vi "Periodic Tasks.vi"(8 "error in":errorcluster) -> ()   [LabVIEW 2015]
doc: "This VI runs in parallel to other tasks. It can contain as many user-defined periodic loops as you need. These can carry out PID or other sorts of timed response."
uses:
  ArmController/Typedef/ArmRef.ctl
  <vilib>/Rock Robotics/WPI/Potentiometer/WPI_PotentiometerDevRef.ctl
  <vilib>/Rock Robotics/SystemInterfaces/AI/FPGA_AIChannel.ctl
  <vilib>/Rock Robotics/WPI/MotorControl/WPI_MotorControlDeviceRef.ctl
  <vilib>/Rock Robotics/WPI/MotorControl/WPI_MotorControlType.ctl
  <vilib>/Rock Robotics/SystemInterfaces/DIO/FPGA_DIOPWMChannel.ctl
  <vilib>/Rock Robotics/WPI/PWM/WPI_PWMDeadband.ctl
  <vilib>/Rock Robotics/WPI/CAN/Jaguar/SubVIs/WPI_CANJaguar_ControlMode.ctl
  <vilib>/Rock Robotics/WPI/CAN/TalonSRX/WPI_CANTalonSRX_APIControlMode.ctl
  ArmController/Typedef/MessageType.ctl
  <vilib>/Rock Robotics/WPI/RobotDrive/WPI_RobotDriveDevRef.ctl
  Typedef/IntakeControllerMsg.ctl
  Typedef/IntakeControllerActions.ctl
  <vilib>/Rock Robotics/WPI/Utilities/WPI_GetSetVariantRefNum.vi
  <vilib>/Rock Robotics/WPI/Power/WPI_Power Get 5Volt Rail Voltage and Current.vi
  <vilib>/Rock Robotics/Network Tables/NT Write Number.vi
  ArmController/ArmController.lvlib
  NavX/navX Library v2.lvlib
panel:
  out "Logger timeout":bool
  out "# elements in Log queue":i32
  in  "Watts Rear":dbl=250.0 format="%#_13g"
  in  "Watts":dbl=320.0 format="%#_13g"
  out "Active Action":string
  in  "?":T1(tab)
  out "Motor Currents":T2(graph)
  out "Motor Power":T3(graph)
  out "Motor Voltage":dbl(graph)
  out "Pressure (psi)":dbl
  out "Pressure":dbl(graph)
  # "Competition: 320"
  # "Competition: 250"
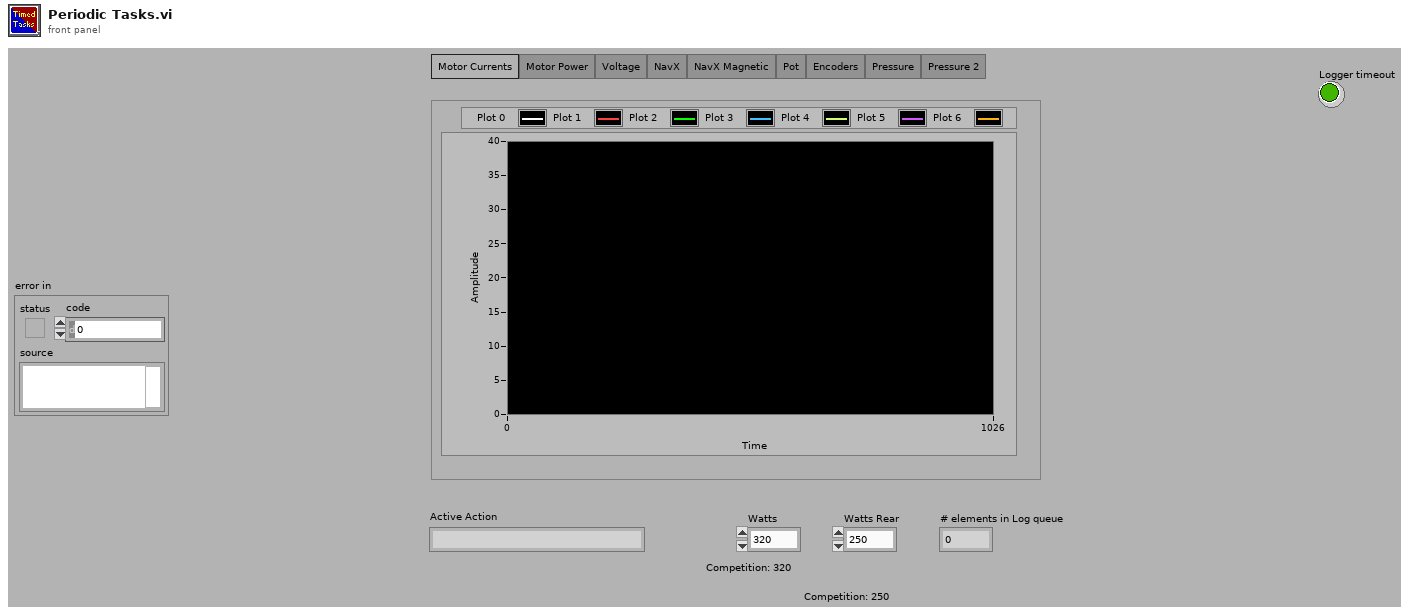
[diagram p1: front panel]
types:
  T1 = enum32{"Motor Currents", "Motor Power", "Voltage", "NavX", "NavX Magnetic", "Pot", "Encoders", "Pressure", "Pressure 2"}
  T2 = cluster{"all currents (A)[0]":dbl, "all currents (A)[1]":dbl, "all currents (A)[2]":dbl, "all currents (A)[3]":dbl, "all currents (A)[4]":dbl, "all currents (A)[5]":dbl, "all currents (A)[6]":dbl, "all currents (A)[7]":dbl, "all currents (A)[8]":dbl, "all currents (A)[9]":dbl, "all currents (A)[10]":dbl, "all currents (A)[11]":dbl, "all currents (A)[12]":dbl, "all currents (A)[13]":dbl}
  T3 = cluster{"[0]":dbl, "[1]":dbl, "[2]":dbl, "[3]":dbl, "[4]":dbl, "[5]":dbl, "[6]":dbl, "[7]":dbl, "[8]":dbl, "[9]":dbl, "[10]":dbl, "[11]":dbl, "[12]":dbl, "[13]":dbl}
  T4 = typedef "ArmController.lvlib/ArmRef.ctl" = cluster{"Pot":T5, "ArmMotor":T7, "Queue":refnum<queue>, "Setpoint":dbl, "Manual":bool, "output range":cluster{"output high":dbl, "output low":dbl}, "PID gains":cluster{"proportional gain (Kc)":dbl, "integral time (Ti, min)":dbl, "derivative time (Td, min)":dbl}}
  T5 = typedef "WPI_PotentiometerDevRef.ctl" = cluster{"DevStatus":errorcluster, "Analog Channel":T6, "Invert Output":bool}
  T6 = typedef "FPGA_AIChannel.ctl" = enum8{"AI 0", "AI 1", "AI 2", "AI 3", "AI MXP 0", "AI MXP 1", "AI MXP 2", "AI MXP 3", "Invalid"}
  T7 = typedef "WPI_MotorControlDeviceRef.ctl" = cluster{"DeviceStatus":errorcluster, "Type":T8, "PWM":cluster{"PWM Channel":T9, "DeadBand":T10}, "CAN":cluster{"Device Number":u8, "Control Mode":T11, "Semaphore":T12, "Max Vout":dbl, "TalonSRX Control Mode":T13}, "Invert":bool}
  T8 = typedef "WPI_MotorControlType.ctl" = enum16{"PWM", "CAN", "CANTalonSRX"}
  T9 = typedef "FPGA_DIOPWMChannel.ctl" = enum8{"PWM 0", "PWM 1", "PWM 2", "PWM 3", "PWM 4", "PWM 5", "PWM 6", "PWM 7", "PWM 8", "PWM 9", "PWM MXP 0", "PWM MXP 1", "PWM MXP 2", "PWM MXP 3", "PWM MXP 4", "PWM MXP 5", "PWM MXP 6", "PWM MXP 7", "PWM MXP 8", "PWM MXP 9", "Invalid"}
  T10 = typedef "WPI_PWMDeadband.ctl" = cluster{"Name":string, "maxPositivePwm":i32, "minPositivePwm":i32, "centerPwm":i32, "maxNegativePwm":i32, "minNegativePwm":i32, "angularRange":u16}
  T11 = typedef "WPI_CANJaguar_ControlMode.ctl" = enum8{"Percent VBus", "Current", "Speed", "Position", "Voltage"}
  T12 = typedef "Semaphore RefNum" = refnum<k1>
  T13 = typedef "WPI_CANTalonSRX_APIControlMode.ctl" = enum8{"Percent VBus", "Speed", "Position", "Slave", "Unchanged / Invalid", "Voltage Compensation", "Current", "Motion Profile"}
  T14 = typedef "WPI_RobotDriveDevRef.ctl" = cluster{"DevStatus":errorcluster, "Motors[]":T7[], "Square Inputs":bool, "Max Output":dbl}
  T15 = cluster{"Front Arm":T4, "Rear Arm":T4, "Front Roller":T7, "Rear Roller":T7, "Drivetrain":T14, "Front Roller":dbl, "Rear Roller":dbl}
  T16 = typedef "WPI_JoystickDevRef.ctl" = cluster{"Device":T17}
  T17 = typedef "WPI_JoystickDeviceEnum.ctl" = enum16{"USB 0", "USB 1", "USB 2", "USB 3", "USB 4", "USB 5"}
  T18 = cluster{"JoystickDevRef":T16, "RobotDriveDevRef":T14}
  T19 = typedef "WPI_SwitchDevRef.ctl" = cluster{"DevStatus":errorcluster, "DIO Channel":T20, "CntIndex":T21, "Normally Closed":bool}
  T20 = typedef "FPGA_DIOChannel.ctl" = enum8{"DIO 0", "DIO 1", "DIO 2", "DIO 3", "DIO 4", "DIO 5", "DIO 6", "DIO 7", "DIO 8", "DIO 9", "DIO MXP 0", "DIO MXP 1", "DIO MXP 2", "DIO MXP 3", "DIO MXP 4", "DIO MXP 5", "DIO MXP 6", "DIO MXP 7", "DIO MXP 8", "DIO MXP 9", "DIO MXP 10", "DIO MXP 11", "DIO MXP 12", "DIO MXP 13", "DIO MXP 14", "DIO MXP 15", "Invalid"}
  T21 = typedef "FPGA_CounterCtrSystemIndex.ctl" = enum8{"Ctr 0", "Ctr 1", "Ctr 2", "Ctr 3", "Ctr 4", "Ctr 5", "Ctr 6", "Ctr 7", "Invalid"}
  T22 = typedef "WPI_AnalogChannelDevRef.ctl" = cluster{"DevStatus":errorcluster, "Analog Channel":T6}
  T23 = typedef "IntakeControllerMsg.ctl" = cluster{"Cmd":T24, "Data":variant}
  T24 = typedef "IntakeControllerActions.ctl" = enum16{"Wait on Intake Rear", "Wait on Angle Rear", "Go To Angle Rear", "Wait on Intake Front", "Wait on Angle Front", "Set Roller Front", "Set Roller Rear", "Go To Angle Front", "Wait ms"}
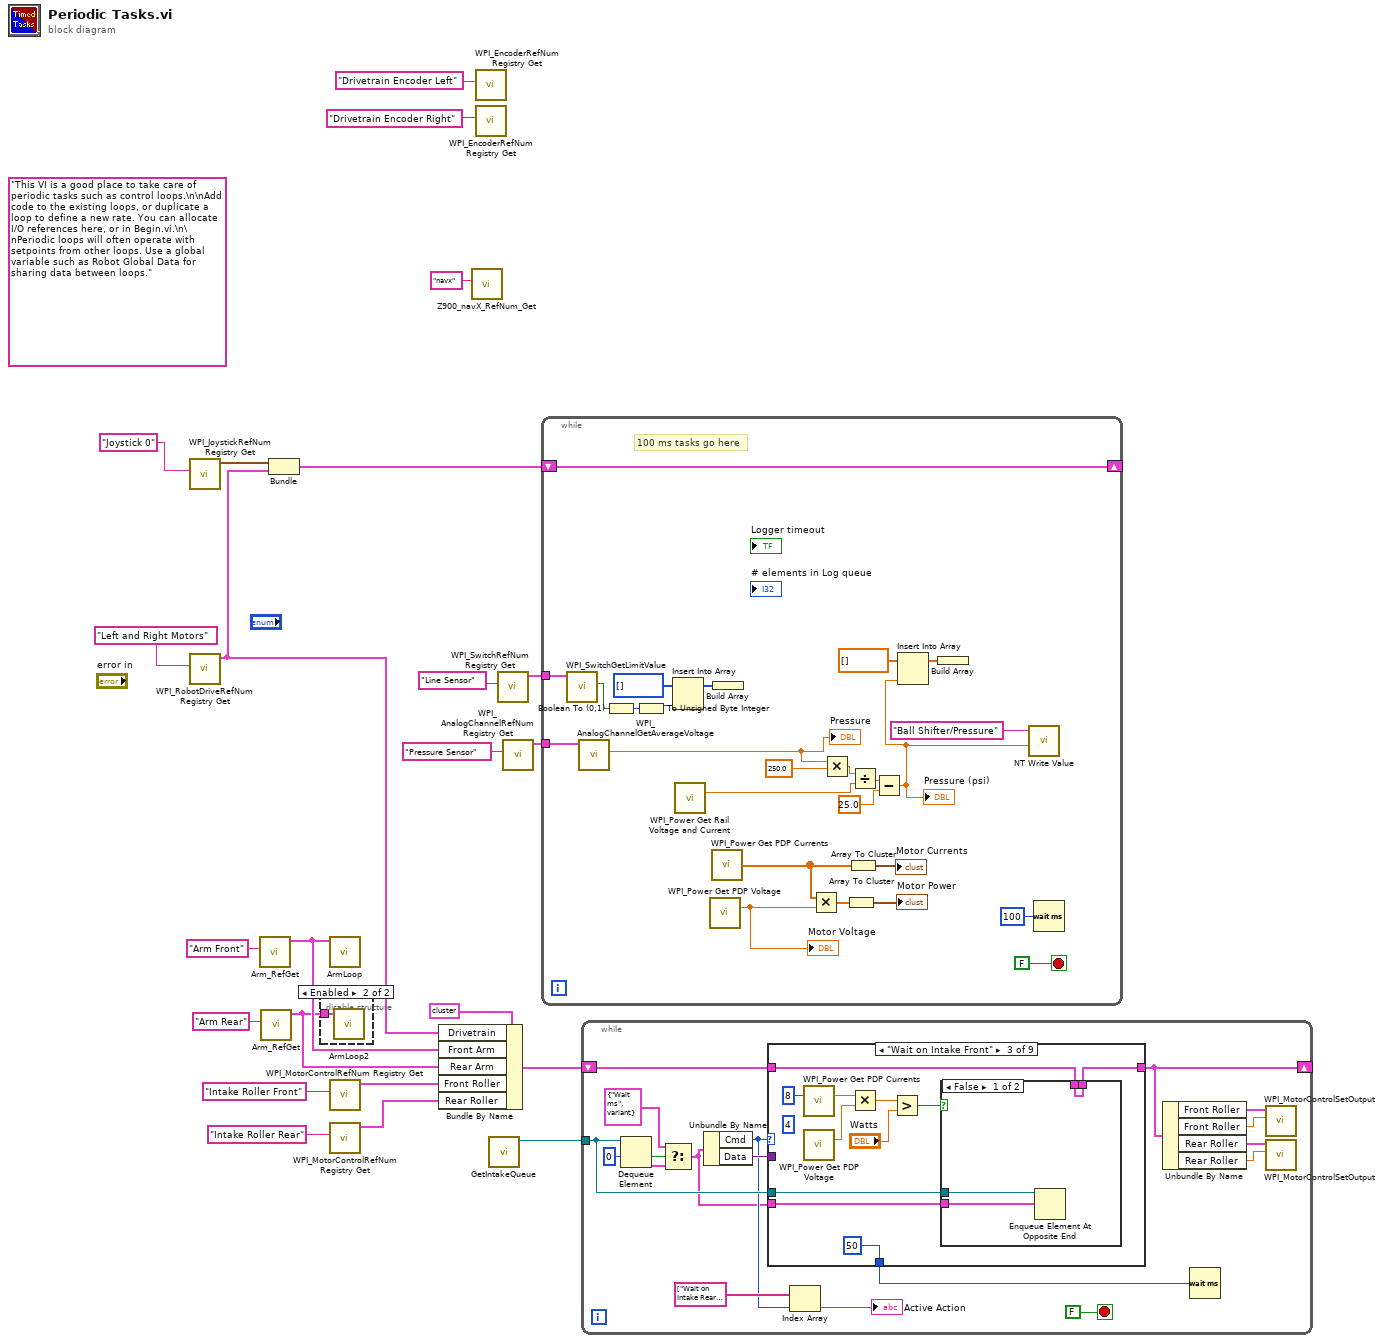
[diagram p0: block diagram]
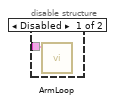
[diagram p2: hidden frame]
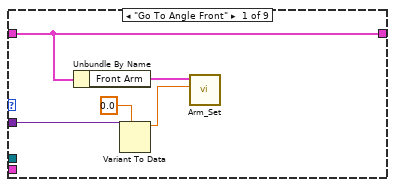
[diagram p3: hidden frame]
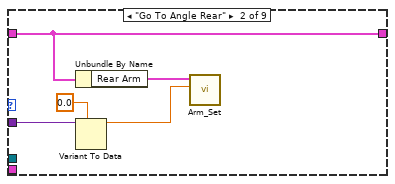
[diagram p4: hidden frame]
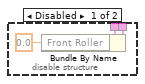
[diagram p6: hidden frame]
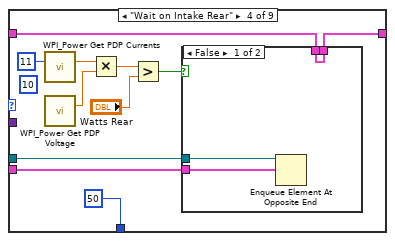
[diagram p7: hidden frame]
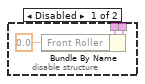
[diagram p9: hidden frame]
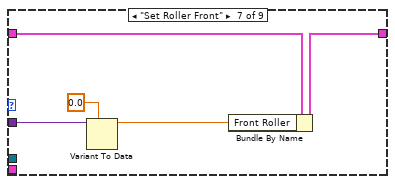
[diagram p12: hidden frame]
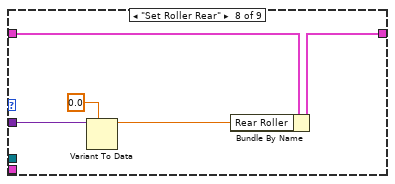
[diagram p13: hidden frame]
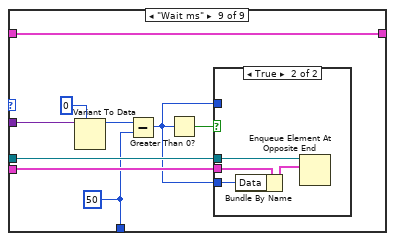
[diagram p14: hidden frame]
diagram:
  (unwired) "This VI is a good place to take care of periodic tasks such as control loops.\n\nAdd code to the existing loops, or duplicate a loop to define a new rate. You can allocate I/O references here, or in Begin.vi.\n\nPeriodic loops will often operate with setpoints from other loops. Use a global variable such as Robot Global Data for sharing data between loops."
  n1 = call <vilib>:"WPI_JoystickRefNum Registry Get.vi"("refnum name"="Joystick 0") -> ("JoystickDevRef"=w21:T16)  [unwired: 1 in, 9 out]
  n2 = call <vilib>:"WPI_RobotDriveRefNum Registry Get.vi"("refnum name"="Left and Right Motors") -> ("RobotDriveDevRef"=w10:T14)  [unwired: 1 in, 9 out]
  n3 = call "Arm_RefGet.vi"("refnum name"="Arm Front") -> ("ArmRef"=w17:T4)  [unwired: 9 in, 1 out]
  n4 = call "Arm_RefGet.vi"("refnum name"="Arm Rear") -> ("ArmRef"=w16:T4)  [unwired: 9 in, 1 out]
  n5 = Bundle("JoystickDevRef"=w21, "RobotDriveDevRef"=w10) -> (w20:T18)  [unwired: 1 out]
  n6 = disable-structure shown="Enabled" {
    disable-tunnel: w16 -> [w24 w25]
    frame Disabled {
      n7 = call "ArmLoop.vi"("ArmRef"=w24) -> ()  [unwired: 11 in]
    }
    frame Enabled {
      n8 = call "ArmLoop2.vi"("ArmRef"=w25) -> ()  [unwired: 11 in]
    }
  }
  n9 = call "ArmLoop.vi"("ArmRef"=w17) -> ()  [unwired: 11 in]
  n10 = call <vilib>:"WPI_MotorControlRefNum Registry Get.vi"("refnum name"="Intake Roller Front") -> ("MotorControlDevRef"=w13:T7)  [unwired: 9 in, 1 out]
  n11 = call <vilib>:"WPI_MotorControlRefNum Registry Get.vi"("refnum name"="Intake Roller Rear") -> ("MotorControlDevRef"=w12:T7)  [unwired: 9 in, 1 out]
  n12 = Bundle By Name(cluster=T15 {"Front Arm"={"Pot"={"DevStatus"={"status"=FALSE, "code"=0, "source"=""}, "Analog Channel"=enum."AI 0", "Invert Output"=FALSE}, "ArmMotor"={"DeviceStatus"={"status"=FALSE, "code"=0, "source"=""}, "Type"=enum."PWM", "PWM"={"PWM Channel"=enum."PWM 0", "DeadBand"={"Name"="", "maxPositivePwm"=0, "minPositivePwm"=0, "centerPwm"=0, "maxNegativePwm"=0, "minNegativePwm"=0, "angularRange"=0}}, "CAN"={"Device Number"=0, "Control Mode"=enum."Percent VBus", "Semaphore"=refnum, "Max Vout"=0.0, "TalonSRX Control Mode"=enum."Percent VBus"}, "Invert"=FALSE}, "Queue"=refnum, "Setpoint"=0.0, "Manual"=FALSE, "output range"={"output high"=0.0, "output low"=0.0}, "PID gains"={"proportional gain (Kc)"=0.0, "integral time (Ti, min)"=0.0, "derivative time (Td, min)"=0.0}}, "Rear Arm"={"Pot"={"DevStatus"={"status"=FALSE, "code"=0, "source"=""}, "Analog Channel"=enum."AI 0", "Invert Output"=FALSE}, "ArmMotor"={"DeviceStatus"={"status"=FALSE, "code"=0, "source"=""}, "Type"=enum."PWM", "PWM"={"PWM Channel"=enum."PWM 0", "DeadBand"={"Name"="", "maxPositivePwm"=0, "minPositivePwm"=0, "centerPwm"=0, "maxNegativePwm"=0, "minNegativePwm"=0, "angularRange"=0}}, "CAN"={"Device Number"=0, "Control Mode"=enum."Percent VBus", "Semaphore"=refnum, "Max Vout"=0.0, "TalonSRX Control Mode"=enum."Percent VBus"}, "Invert"=FALSE}, "Queue"=refnum, "Setpoint"=0.0, "Manual"=FALSE, "output range"={"output high"=0.0, "output low"=0.0}, "PID gains"={"proportional gain (Kc)"=0.0, "integral time (Ti, min)"=0.0, "derivative time (Td, min)"=0.0}}, "Front Roller"={"DeviceStatus"={"status"=FALSE, "code"=0, "source"=""}, "Type"=enum."PWM", "PWM"={"PWM Channel"=enum."Invalid", "DeadBand"={"Name"="", "maxPositivePwm"=0, "minPositivePwm"=0, "centerPwm"=0, "maxNegativePwm"=0, "minNegativePwm"=0, "angularRange"=0}}, "CAN"={"Device Number"=0, "Control Mode"=enum."Percent VBus", "Semaphore"=refnum, "Max Vout"=12.0, "TalonSRX Control Mode"=enum."Percent VBus"}, "Invert"=FALSE}, "Rear Roller"={"DeviceStatus"={"status"=FALSE, "code"=0, "source"=""}, "Type"=enum."PWM", "PWM"={"PWM Channel"=enum."Invalid", "DeadBand"={"Name"="", "maxPositivePwm"=0, "minPositivePwm"=0, "centerPwm"=0, "maxNegativePwm"=0, "minNegativePwm"=0, "angularRange"=0}}, "CAN"={"Device Number"=0, "Control Mode"=enum."Percent VBus", "Semaphore"=refnum, "Max Vout"=12.0, "TalonSRX Control Mode"=enum."Percent VBus"}, "Invert"=FALSE}, "Drivetrain"={"DevStatus"={"status"=FALSE, "code"=0, "source"=""}, "Motors[]"=[], "Square Inputs"=FALSE, "Max Output"=1.0}, "Front Roller"=0.0, "Rear Roller"=0.0}, "Drivetrain"=w10, "Front Arm"=w17, "Rear Arm"=w16, "Front Roller"=w13, "Rear Roller"=w12) -> (w18:T15)
  n13 = call "Z900_navX_RefNum_Get.vi"("refnum name"="navx") -> ()  [unwired: 9 in, 2 out]
  n14 = call <vilib>:"WPI_EncoderRefNum Registry Get.vi"("refnum name"="Drivetrain Encoder Left") -> ()  [unwired: 9 in, 2 out]
  n15 = call <vilib>:"WPI_EncoderRefNum Registry Get.vi"("refnum name"="Drivetrain Encoder Right") -> ()  [unwired: 9 in, 2 out]
  n16 = call "GetIntakeQueue.vi"() -> ("queue out"=w11:refnum<queue>)  [unwired: 11 in]
  n17 = call <vilib>:"WPI_SwitchRefNum Registry Get.vi"("refnum name"="Line Sensor") -> ("SwitchDevRef"=w4:T19)  [unwired: 9 in, 1 out]
  n18 = call <vilib>:"WPI_AnalogChannelRefNum Registry Get.vi"("refnum name"="Pressure Sensor") -> ("AIDeviceRef"=w6:T22)  [unwired: 9 in, 1 out]
  n19 = while {
    shift-right: [w48] -> _
    shift-left: w20 -> [w48]
    tunnel: w6 -> [w42]
    tunnel: w4 -> [w31]
    stop <- FALSE stop-if-true
    # "100 ms tasks go here"
    n20 = call <vilib>:"WPI_SwitchGetLimitValue.vi"("SwitchDevRef"=w31) -> ("Switch Pressed"=w28:bool)  [unwired: 8 in, 2 out]
    n21 = call <vilib>:"WPI_AnalogChannelGetAverageVoltage.vi"("AIDeviceRef"=w42) -> ("Voltage"=w40:dbl)  [unwired: 8 in, 2 out]
    "Pressure" <- w40
    n22 = Boolean To (0,1)(Boolean=w28) -> (0, 1=w27:i16)
    n23 = To Unsigned Byte Integer(number=w27) -> (unsigned 8bit integer=w26:u8)
    n24 = Insert Into Array(array=u8[] [], new element=w26) -> (w30:u8[])  [unwired: 1 in]
    n25 = call-poly <vilib>:"WPI_Power Get Rail Voltage and Current.vi"() -> ("5 volt rail voltage (V)"=w38:dbl)  [unwired: 13 in, 2 out]
    n26 = call <vilib>:"WPI_Power Get PDP Voltage.vi"() -> ("voltage (V)"=w44:dbl)  [unwired: 14 in, 1 out]
    "Motor Voltage" <- w44
    n27 = call <vilib>:"WPI_Power Get PDP Currents.vi"() -> ("all currents (A)"=w43:dbl[])  [unwired: 13 in, 2 out]
    n28 = Build Array(w30) -> ()  [unwired: 1 out]
    n29 = Multiply(x=w43, y=w44) -> (x*y=w47:dbl[])
    n30 = Multiply(x=w40, y=250.0) -> (x*y=w35:dbl)
    n31 = Array To Cluster(array=w47) -> (cluster=→"Motor Power":T3)
    n32 = Array To Cluster(array=w43) -> (cluster=→"Motor Currents":T2)
    n33 = Divide(x=w35, y=w38) -> (x/y=w36:dbl)
    n34 = Subtract(x=w36, y=25.0) -> (x-y=w34:dbl)
    "Pressure (psi)" <- w34
    n35 = Insert Into Array(array=dbl[] [], new element=w34) -> (w33:dbl[])  [unwired: 1 in]
    n36 = Build Array(w33) -> ()  [unwired: 1 out]
    n37 = call-poly <vilib>:"NT Write Value.vi"("Numeric"=w34, "Name"="Ball Shifter/Pressure") -> ()  [unwired: 9 in, 1 out]
    n38 = Wait (ms)(milliseconds to wait=u32 100) -> ()  [unwired: 1 out]
  }
  n39 = while {
    shift-right: [w62] -> _
    shift-left: w18 -> [w68]
    tunnel: w11 -> [w63]
    stop <- FALSE stop-if-true
    n40 = Dequeue Element(queue=w63, timeout in ms (-1)=0) -> (element=w56:T23, timed out?=w57:bool)  [unwired: 1 in, 2 out]
    n41 = Select(t=T23 {"Cmd"=enum."Wait ms", "Data"=variant(i32 50)} ("output cluster"), s=w57, f=w56) -> (s? t:f=w52:T23)
    n42 = Unbundle By Name(w52) -> ("Cmd"=w54:T24, "Data"=w66:variant)
    n43 = case shown="\"Wait on Intake Front\"" w54 {
      tunnel: w68 -> [w73 w78 w88 w108 w119 w120 w123 w128 w139]
      tunnel: [w73 w78 w87 w107 w119 w120 w122 w127 w139] -> w62
      tunnel: w66 -> [w70 w76 _ _ _ _ w124 w129 w137]
      tunnel: w63 -> [_ _ w89 w109 _ _ _ _ w134]
      tunnel: w52 -> [_ _ w86 w106 _ _ _ _ w133]
      tunnel: [_ _ u32 50 ("milliseconds to wait") u32 50 ("milliseconds to wait") _ _ _ _ w131] -> w51
      frame "Go To Angle Front" {
        n44 = Unbundle By Name(w73) -> ("Front Arm"=w72:T4)
        n45 = Variant To Data(type=0.0, Variant=w70) -> (data=w69:dbl)  [unwired: 1 in, 1 out]
        n46 = call "Arm_Set.vi"("Value"=w69, "ArmRef in"=w72) -> ()  [unwired: 8 in, 2 out]
      }
      frame "Go To Angle Rear" {
        n47 = Unbundle By Name(w78) -> ("Rear Arm"=w77:T4)
        n48 = Variant To Data(type=0.0, Variant=w76) -> (data=w74:dbl)  [unwired: 1 in, 1 out]
        n49 = call "Arm_Set.vi"("Value"=w74, "ArmRef in"=w77) -> ()  [unwired: 8 in, 2 out]
      }
      frame "Wait on Intake Front" {
        (unwired) 4 ("PDP Channel")
        n50 = call <vilib>:"WPI_Power Get PDP Currents.vi"("PDP Channel"=8) -> ("current (A)"=w82:dbl)  [unwired: 12 in, 2 out]
        n51 = call <vilib>:"WPI_Power Get PDP Voltage.vi"() -> ("voltage (V)"=w80:dbl)  [unwired: 14 in, 1 out]
        n52 = Multiply(x=w82, y=w80) -> (x*y=w83:dbl)
        n53 = Greater?(x=w83, y="Watts") -> (0:w85:bool)
        n54 = case shown="False" w85 {
          tunnel: w89 -> [w91 _]
          tunnel: w88 -> [w92 w94]
          tunnel: [w92 w93] -> w87
          tunnel: w86 -> [w90 _]
          frame False {
            n55 = Enqueue Element At Opposite End(queue=w91, element=w90) -> ()  [unwired: 2 in, 3 out]
          }
          frame True {
            n56 = disable-structure shown="Enabled" {
              disable-tunnel: w94 -> [w97 w98]
              disable-tunnel: [w95 w98] -> w93
              frame Disabled {
                n57 = Bundle By Name(cluster=w97, "Front Roller"=0.0) -> (w95:T15)
              }
              frame Enabled {
              }
            }
          }
        }
      }
      frame "Wait on Intake Rear" {
        (unwired) 10 ("PDP Channel")
        n58 = call <vilib>:"WPI_Power Get PDP Currents.vi"("PDP Channel"=11) -> ("current (A)"=w102:dbl)  [unwired: 12 in, 2 out]
        n59 = call <vilib>:"WPI_Power Get PDP Voltage.vi"() -> ("voltage (V)"=w100:dbl)  [unwired: 14 in, 1 out]
        n60 = Multiply(x=w102, y=w100) -> (x*y=w103:dbl)
        n61 = Greater?(x=w103, y="Watts Rear") -> (0:w105:bool)
        n62 = case shown="False" w105 {
          tunnel: w109 -> [w111 _]
          tunnel: w108 -> [w112 w114]
          tunnel: [w112 w113] -> w107
          tunnel: w106 -> [w110 _]
          frame False {
            n63 = Enqueue Element At Opposite End(queue=w111, element=w110) -> ()  [unwired: 2 in, 3 out]
          }
          frame True {
            n64 = disable-structure shown="Enabled" {
              disable-tunnel: w114 -> [w117 w118]
              disable-tunnel: [w115 w118] -> w113
              frame Disabled {
                n65 = Bundle By Name(cluster=w117, "Front Roller"=0.0) -> (w115:T15)
              }
              frame Enabled {
              }
            }
          }
        }
      }
      frame "Wait on Angle Front" {
      }
      frame "Wait on Angle Rear" {
      }
      frame "Set Roller Front" {
        n66 = Variant To Data(type=0.0, Variant=w124) -> (data=w121:dbl)  [unwired: 1 in, 1 out]
        n67 = Bundle By Name(cluster=w123, "Front Roller"=w121) -> (w122:T15)
      }
      frame "Set Roller Rear" {
        n68 = Variant To Data(type=0.0, Variant=w129) -> (data=w126:dbl)  [unwired: 1 in, 1 out]
        n69 = Bundle By Name(cluster=w128, "Rear Roller"=w126) -> (w127:T15)
      }
      frame "Wait ms" {
        w131 = u32 50 ("milliseconds to wait")
        n70 = Variant To Data(type=u32 0, Variant=w137) -> (data=w136:u32)  [unwired: 1 in, 1 out]
        n71 = Subtract(x=w136, y=w131) -> (x-y=w132:u32)
        n72 = Greater Than 0?(x=w132) -> (x > 0?=w135:bool)
        n73 = case shown="True" w135 {
          tunnel: w132 -> [_ _]
          tunnel: w134 -> [_ w143]
          tunnel: w133 -> [_ w142]
          tunnel: w132 -> [_ w141]
          frame False {
          }
          frame True {
            n74 = Bundle By Name(cluster=w142, "Data"=w141) -> (w140:T23)
            n75 = Enqueue Element At Opposite End(queue=w143, element=w140) -> ()  [unwired: 2 in, 3 out]
          }
        }
      }
    }
    n76 = Index Array(array=string[] ["Wait on Intake Rear", "Wait on Intake Rear", "Wait on Intake Rear", "Wait on Intake Rear", "Wait on Intake Rear", "Wait on Intake Rear", "Wait on Intake Rear"] ("Array"), index=w54) -> (element=→"Active Action":string)
    n77 = Unbundle By Name(w62) -> ("Front Roller"=w61:T7, "Front Roller"=w60:dbl, "Rear Roller"=w58:T7, "Rear Roller"=w59:dbl)
    n78 = Wait (ms)(milliseconds to wait=w51) -> ()  [unwired: 1 out]
    n79 = call <vilib>:"WPI_MotorControlSetOutput.vi"("Output"=w60, "MotorControlDevRef"=w61) -> ()  [unwired: 7 in, 3 out]
    n80 = call <vilib>:"WPI_MotorControlSetOutput.vi"("Output"=w59, "MotorControlDevRef"=w58) -> ()  [unwired: 7 in, 3 out]
  }
